vi "uc480_SubVI_Example_Flash.vi"(0 ".NET (Reference)":refnum<k24>, 5 "Flash Mode":u8, 7 "Flash Duration":u32, 9 "Flash Delay":u32, 11 "Fehler":errorcluster caption="Error In") -> (4 "Delay":u32, 6 "Duration":u32, 15 "Error":errorcluster caption="Error Out")   [LabVIEW 2011]
uses:
  C:/Program Files/Thorlabs/Scientific Imaging/DCx Camera Support/Develop/DotNet/uc480DotNet.dll
  Develop/DotNet/uc480DotNet.dll
  C:/Program Files/IDS/uEye/OtherDrivers/LabVIEW/ueye.NET/uEyeDotNet.dll
  IDS/uEye/OtherDrivers/LabVIEW/ueye.NET/uEyeDotNet.dll
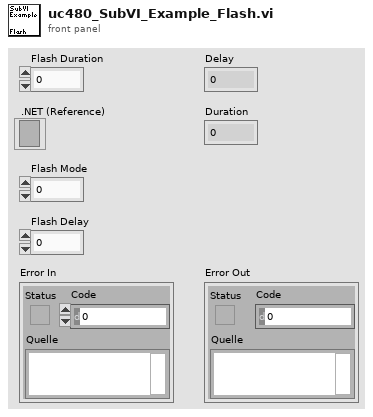
[diagram p1: front panel]
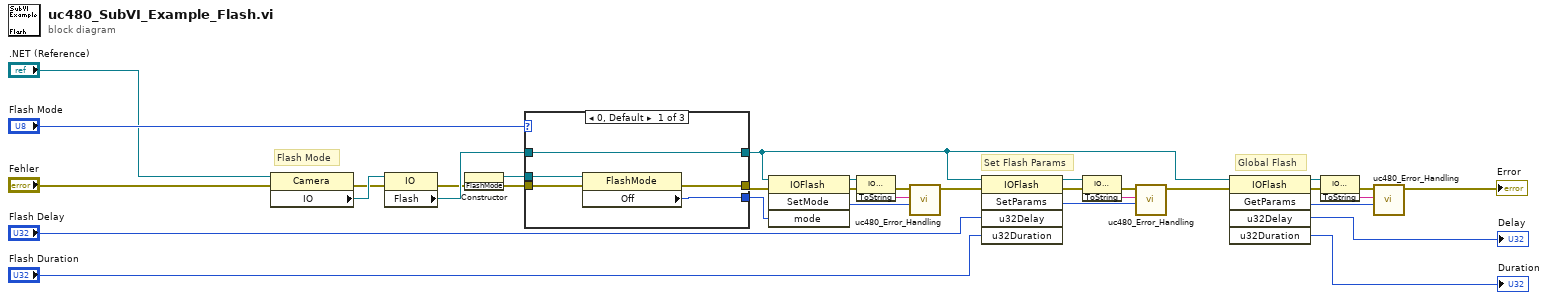
[diagram p0: block diagram]
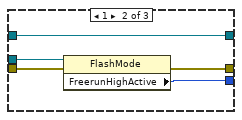
[diagram p2: hidden frame]
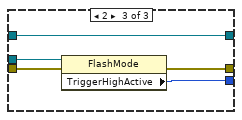
[diagram p3: hidden frame]
diagram:
  # "Global Flash"
  # "Set Flash Params"
  # "Flash Mode"
  n1 = property on="Eigenschaftsknoten" class="Camera"(reference=".NET (Reference)", error in="Fehler") -> (error out=w3:errorcluster, "IO"=w4:refnum<k24>)  [unwired: 1 out]
  n2 = property on="Eigenschaftsknoten" class="IO"(reference=w4, error in=w3) -> (error out=w1:errorcluster, "Flash"=w22:refnum<k24>)  [unwired: 1 out]
  n3 = constructor class="FlashMode"(error in=w1) -> (reference out=w19:refnum<k24>, error out=w20:errorcluster)  [unwired: 2 in, 1 out]
  n4 = case shown="0, Default" "Flash Mode" {
    tunnel: w19 -> [w39 w43 w48]
    tunnel: w20 -> [w38 w42 w47]
    tunnel: w22 -> [w37 w44 w49]
    tunnel: [w37 w44 w49] -> w25
    tunnel: [w36 w40 w46] -> w21
    tunnel: [w35 w41 w45] -> w2
    frame 0, Default {
      n5 = property class="FlashMode"(reference=w39, error in=w38) -> (error out=w36:errorcluster, "Off"=w35:i32)  [unwired: 1 out]
    }
    frame 1 {
      n6 = property class="FlashMode"(reference=w43, error in=w42) -> (error out=w40:errorcluster, "FreerunHighActive"=w41:i32)  [unwired: 1 out]
    }
    frame 2 {
      n7 = property class="FlashMode"(reference=w48, error in=w47) -> (error out=w46:errorcluster, "TriggerHighActive"=w45:i32)  [unwired: 1 out]
    }
  }
  n8 = invoke class="IOFlash" method="SetMode"(reference=w25, error in=w21, "mode"=w2) -> (reference out=w11:refnum<k24>, error out=w10:errorcluster, "SetMode"=w9:i32)  [unwired: 1 in, 1 out]
  n9 = invoke class="IOFlash" method="ToString"(reference=w11, error in=w10) -> (error out=w7:errorcluster, "ToString"=w8:string)  [unwired: 1 in, 1 out]
  n10 = call "uc480_Error_Handling.vi"("Error Code"=w9, "Error String"=w8, "Error In"=w7) -> ("Error Out"=w12:errorcluster)  [unwired: 8 in]
  n11 = invoke class="IOFlash" method="SetParams"(reference=w25, error in=w12, "u32Delay"="Flash Delay", "u32Duration"="Flash Duration") -> (reference out=w15:refnum<k24>, error out=w16:errorcluster, "SetParams"=w17:i32)  [unwired: 1 in, 2 out]
  n12 = invoke class="IOFlash" method="ToString"(reference=w15, error in=w16) -> (error out=w13:errorcluster, "ToString"=w14:string)  [unwired: 1 in, 1 out]
  n13 = call "uc480_Error_Handling.vi"("Error Code"=w17, "Error String"=w14, "Error In"=w13) -> ("Error Out"=w26:errorcluster)  [unwired: 8 in]
  n14 = invoke class="IOFlash" method="GetParams"(reference=w25, error in=w26) -> (reference out=w31:refnum<k24>, error out=w32:errorcluster, "GetParams"=w34:i32, "u32Delay"=→"Delay":u32, "u32Duration"=→"Duration":u32)  [unwired: 3 in]
  n15 = invoke class="IOFlash" method="ToString"(reference=w31, error in=w32) -> (error out=w29:errorcluster, "ToString"=w30:string)  [unwired: 1 in, 1 out]
  n16 = call "uc480_Error_Handling.vi"("Error Code"=w34, "Error String"=w30, "Error In"=w29) -> ("Error Out"=→"Error":errorcluster)  [unwired: 8 in]
